vi "Data acquisition and analysis.vi"() -> ()   [LabVIEW 2013]
uses:
  DAQ_global.vi
  <vilib>/express/express analysis/Spectral/Block/exnSpectralBlock spectral measurements peak poly.vi
  <vilib>/express/express analysis/Spectral/Block/exnSpectralBlock spectral measurements peak DDT.vi
  <vilib>/express/express analysis/Spectral/XNode/ExpressSpectralMeasurementsBlockNode.xnode
panel:
  out "RMS":dynamicdata(graph)
  out "Spectrum":dynamicdata(graph)
  out "Waveform":dynamicdata(graph) caption="data"
  out "THD":dbl
  out "Frequency":dbl
  out "Amplitude":dbl
  in  "number of samples":i32
  in  "rate":dbl
  in  "stop":bool
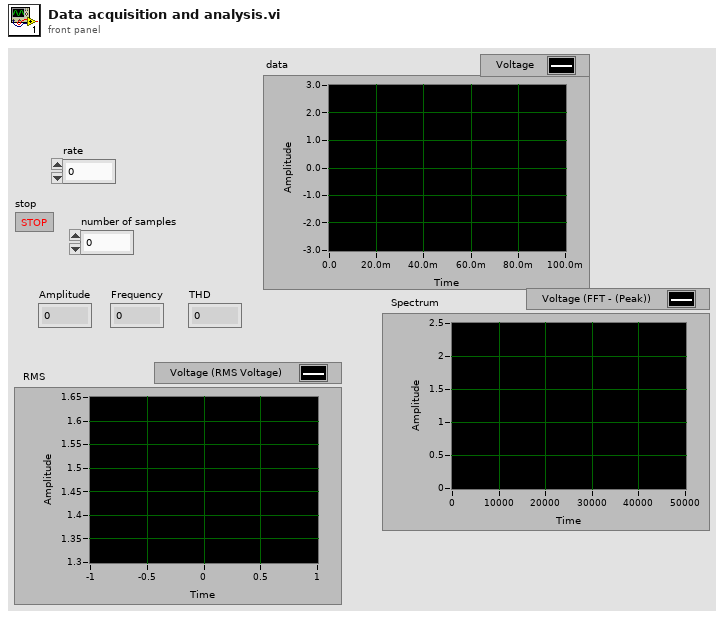
[diagram p1: front panel]
types:
  T1 = cluster{"averaging mode":u16, "weighting mode":u16, "number of averages":u32}
  T2 = cluster{"dB On (F)":bool, "unwrap phase (F)":bool, "convert to degree (F)":bool}
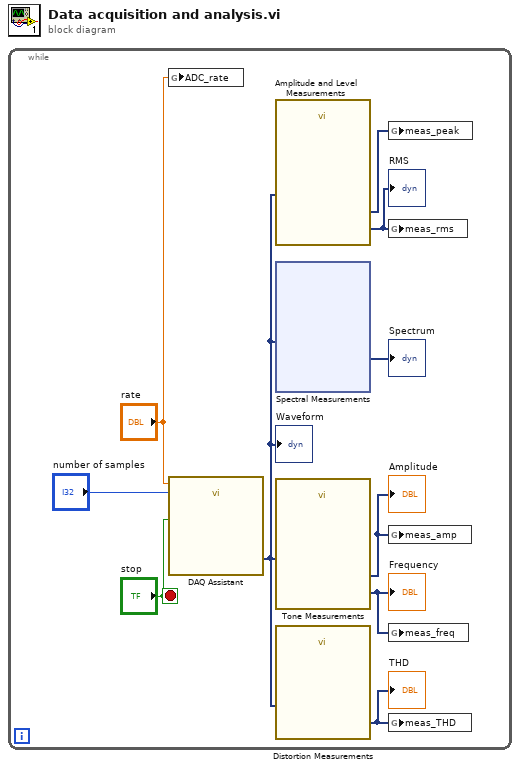
[diagram p0: block diagram]
diagram:
  n1 = while {
    stop <- "stop" stop-if-true
    n2 = global write "DAQ_global.vi" "ADC_rate"("rate") -> ()
    n3 = call "DAQ Assistant"("rate"="rate", "number of samples"="number of samples", "stop (T)"="stop") -> ("data"=w3:dynamicdata)  [unwired: 14 in, 2 out]
    "Waveform" <- w3
    n4 = call "Amplitude and Level Measurements"("Signals"=w3) -> ("RMS"=w2:dynamicdata, "Positive Peak"=w1:dynamicdata)  [unwired: 12 in, 1 out]
    "RMS" <- w2
    n5 = xnode "Spectral Measurements"("Signals"=w3) -> ("FFT - (Peak)"=→"Spectrum":dynamicdata)  [unwired: 1 in, 2 out]
    n6 = call "Tone Measurements"("Signals"=w3) -> ("Frequency"=w5:dynamicdata, "Amplitude"=w6:dynamicdata)  [unwired: 8 in, 1 out]
    "Amplitude" <- w6
    "Frequency" <- w5
    n7 = call "Distortion Measurements"("Signals"=w3) -> ("THD"=w4:dynamicdata)  [unwired: 9 in, 1 out]
    "THD" <- w4
    n8 = global write "DAQ_global.vi" "meas_peak"(w1) -> ()
    n9 = global write "DAQ_global.vi" "meas_rms"(w2) -> ()
    n10 = global write "DAQ_global.vi" "meas_amp"(w6) -> ()
    n11 = global write "DAQ_global.vi" "meas_freq"(w5) -> ()
    n12 = global write "DAQ_global.vi" "meas_THD"(w4) -> ()
  }
